vi "RFH-View-simple_common_selector.vi"() -> ()   [LabVIEW 2020, in "RFH-Reflection_File_Handler.lvlib"]
uses:
  RFH-Reflection_File_Handler.lvlib
panel:
  out "Reflection Imag 2":T1(graph)
  in  "stop":bool
  out "Numeric":i32
  out "Reflection Imag":T1(graph)
  in  "Folder Path":path=path "C:/projects/Universitet/Master/data/Real Test - First libreVNA test with calibration file/Converted Data"
  out "Reflection Real":T1(graph)
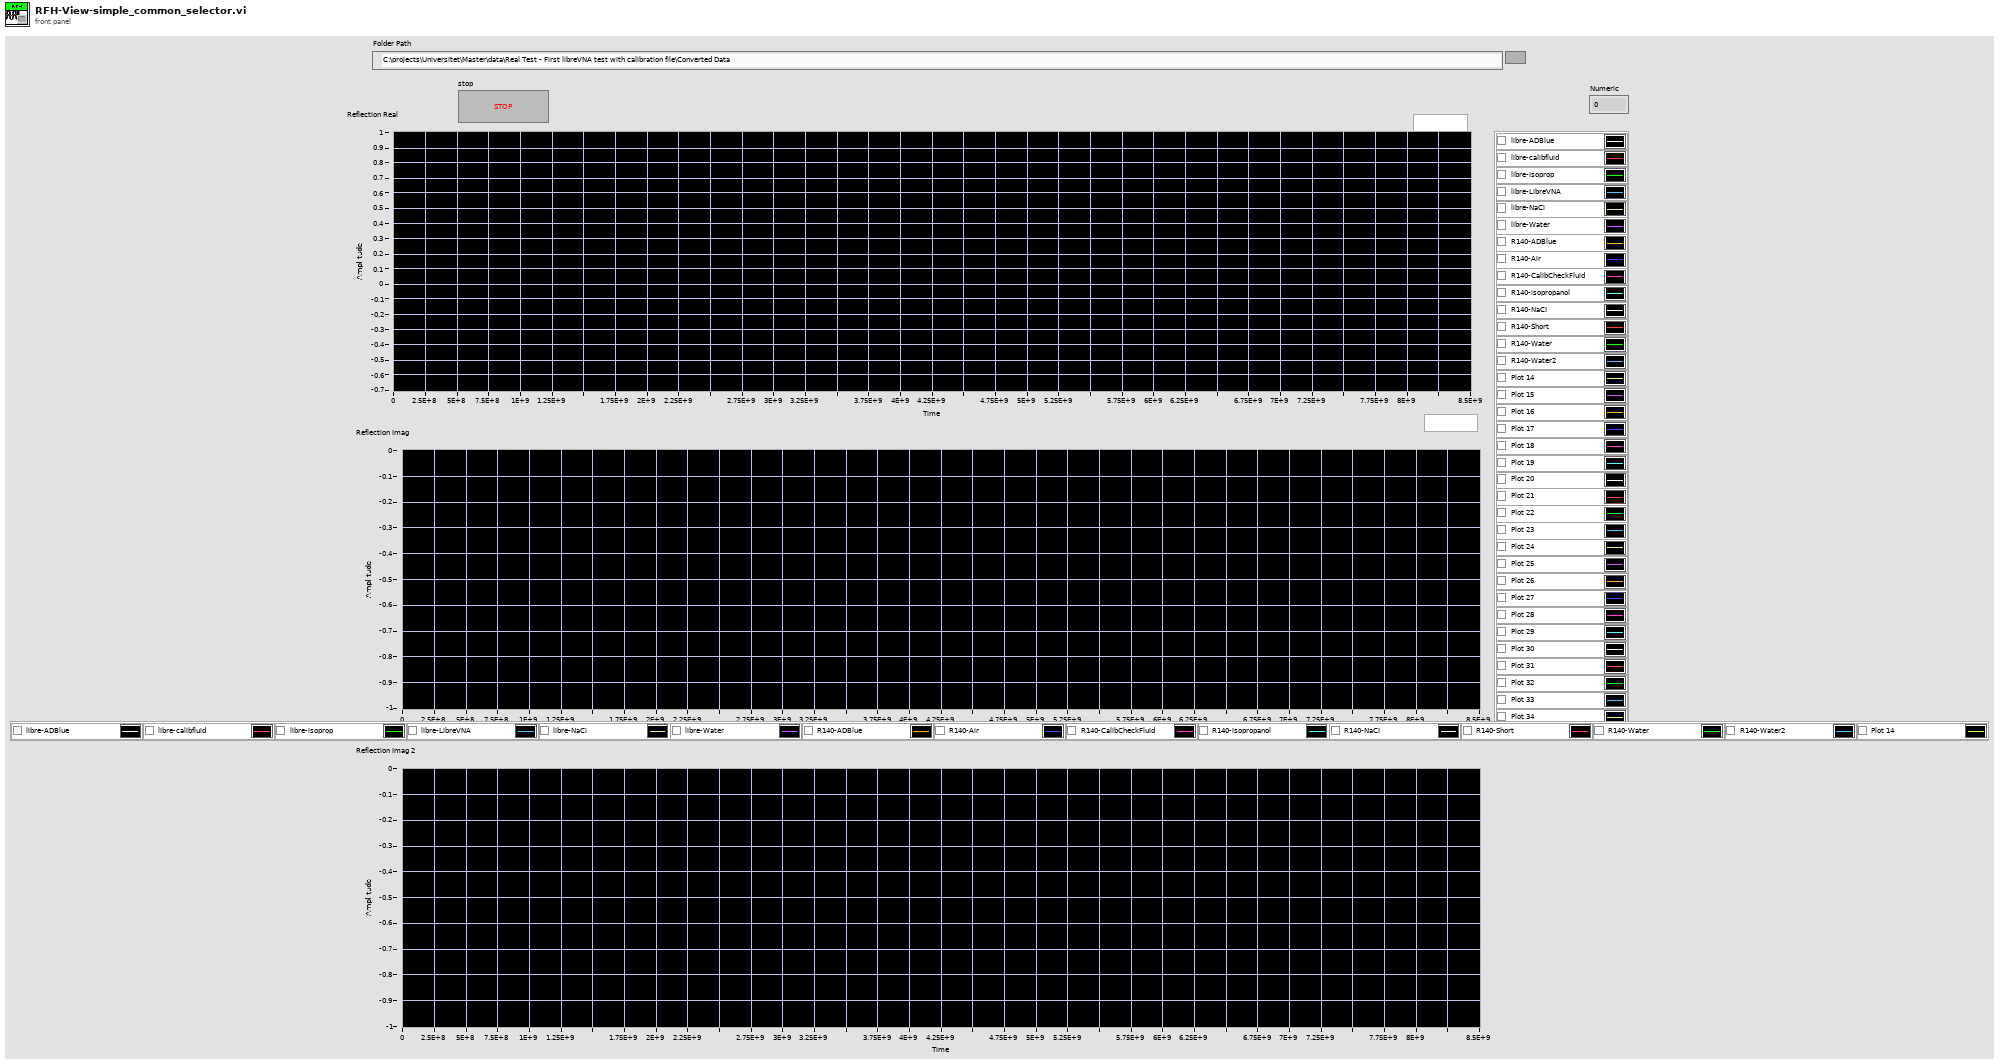
[diagram p1: front panel]
types:
  T1 = cluster{"Frequency":dbl[], "Reflection'":dbl[]}[]
  T2 = typedef "RFH-Reflection_File_Handler.lvlib/RFH-common_data_format.ctl" = cluster{"Frequency":dbl[], "Reflection'":dbl[], "Reflection''":dbl[], "Permativity'":dbl[], "Permativity''":dbl[]}
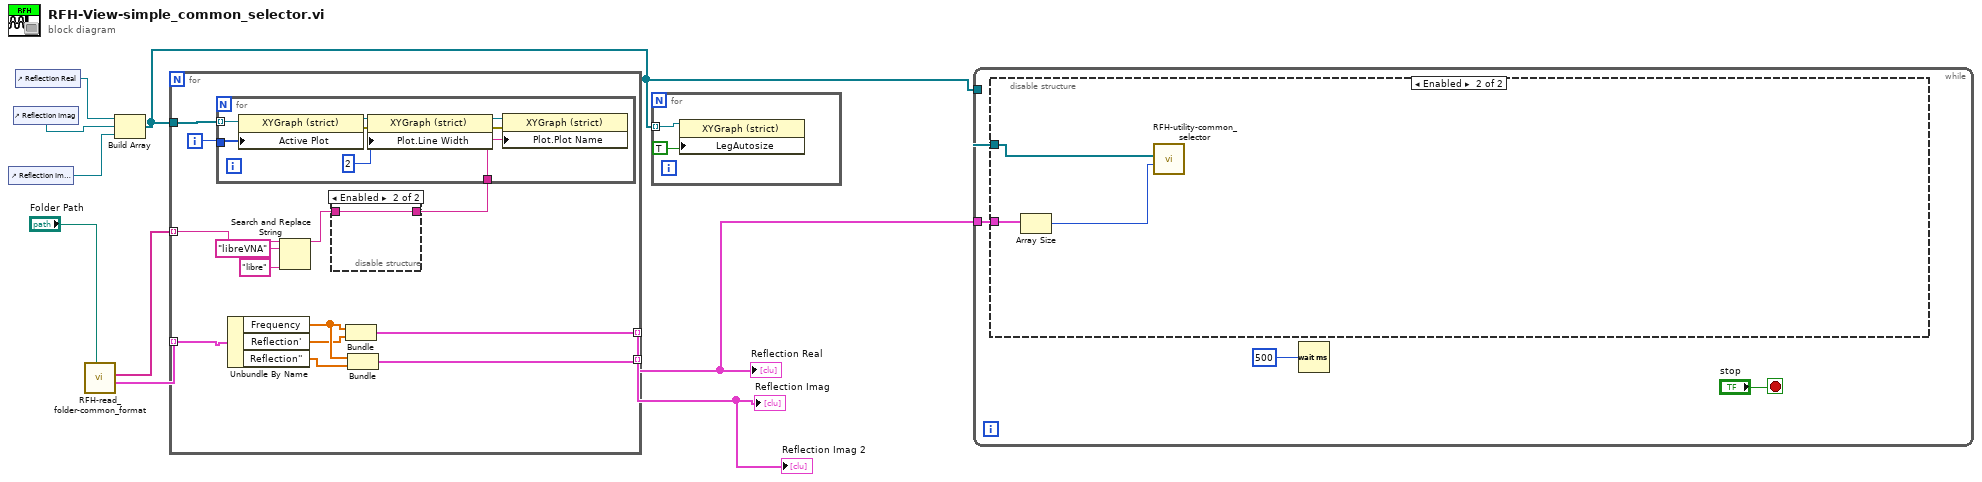
[diagram p0: block diagram]
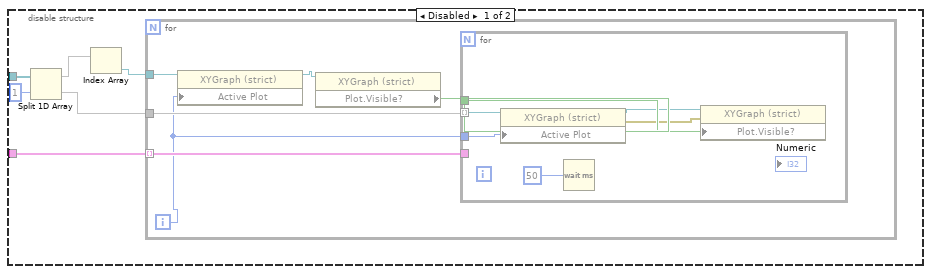
[diagram p2: hidden frame]
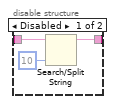
[diagram p3: hidden frame]
diagram:
  n1 = control-ref of="Reflection Imag 2"() -> (w4:refnum<vi>)
  n2 = control-ref of="Reflection Imag"() -> (w2:refnum<vi>)
  n3 = control-ref of="Reflection Real"() -> (w3:refnum<vi>)
  n4 = call "RFH-read_folder-common_format.vi"("Folder Path"="Folder Path") -> ("Data"=w9:T2[], "Names"=w7:string[])  [unwired: 8 in, 1 out]
  n5 = Build Array(w3, w2, w4) -> (w6:refnum<vi>[])
  n6 = for {
    tunnel: w9 -> [w22] mode=indexing
    tunnel: [w18] -> w1 mode=indexing
    tunnel: [w17] -> w5 mode=indexing
    tunnel: w7 -> [w14] mode=indexing
    tunnel: w6 -> [w10]
    i -> [w16]
    n7 = Unbundle By Name(w22) -> ("Frequency"=w21:dbl[], "Reflection'"=w20:dbl[], "Reflection''"=w19:dbl[])
    n8 = Search and Replace String(input string=w14, search string="libreVNA", replace string="libre" ("replace string (\"\")")) -> (result string=w11:string)  [unwired: 5 in, 3 out]
    n9 = disable-structure shown="Enabled" {
      disable-tunnel: [w24 w26] -> w15
      disable-tunnel: w11 -> [w23 w26]
      frame Disabled {
        n10 = Search/Split String(string=w23, offset (0)=10) -> (substring before match=w24:string)  [unwired: 1 in, 2 out]
      }
      frame Enabled {
      }
    }
    n11 = for {
      tunnel: w16 -> [w33]
      tunnel: w15 -> [w30]
      tunnel: w10 -> [w29] mode=indexing
      n12 = property on="Property Node" class="XYGraph (strict)"(reference=w29, "Active Plot"=w33) -> (reference out=w28:refnum<vi>, error out=w34:errorcluster)  [unwired: 1 in]
      n13 = property on="Property Node" class="XYGraph (strict)"(reference=w28, error in=w34, "Plot.Line Width"=u8 2) -> (reference out=w27:refnum<vi>, error out=w32:errorcluster)
      n14 = property on="Property Node" class="XYGraph (strict)"(reference=w27, error in=w32, "Plot.Plot Name"=w30) -> ()  [unwired: 2 out]
    }
    n15 = Bundle("Frequency"=w21, "Reflection'"=w20) -> (w18:cluster{"Frequency":dbl[], "Reflection'":dbl[]})  [unwired: 1 in]
    n16 = Bundle("Frequency"=w21, "Reflection''"=w19) -> (w17:cluster{"Frequency":dbl[], "Reflection''":dbl[]})  [unwired: 1 in]
  }
  "Reflection Real" <- w1
  "Reflection Imag" <- w5
  "Reflection Imag 2" <- w5
  n17 = for {
    tunnel: w6 -> [w35] mode=indexing
    n18 = property on="Property Node" class="XYGraph (strict)"(reference=w35, "LegAutosize"=TRUE ("Legend:Autosize")) -> ()  [unwired: 1 in, 2 out]
  }
  n19 = while {
    tunnel: w6 -> [w40]
    tunnel: w1 -> [w38]
    stop <- "stop" stop-if-true
    n20 = disable-structure shown="Enabled" {
      disable-tunnel: w40 -> [w46 w61]
      disable-tunnel: w38 -> [w42 w60]
      frame Disabled {
        n21 = Split 1D Array(array=w46, index=1) -> (first subarray=w44:refnum<vi>[], second subarray=w43:refnum<vi>[])
        n22 = Index Array(array=w44) -> (element=w41:refnum<vi>)  [unwired: 1 in]
        n23 = for {
          tunnel: w43 -> [w52]
          tunnel: w42 -> [w50] mode=indexing
          tunnel: w41 -> [w49]
          i -> [w47]
          n24 = property on="Property Node" class="XYGraph (strict)"(reference=w49, "Active Plot"=w47) -> (reference out=w48:refnum<vi>)  [unwired: 1 in, 1 out]
          n25 = property on="Property Node" class="XYGraph (strict)"(reference=w48) -> ("Plot.Visible?"=w51:bool)  [unwired: 1 in, 2 out]
          n26 = for {
            tunnel: w51 -> [w58]
            tunnel: w52 -> [w57] mode=indexing
            tunnel: w50 -> [_]
            tunnel: w47 -> [w53]
            n27 = property on="Property Node" class="XYGraph (strict)"(reference=w57, "Active Plot"=w53) -> (reference out=w56:refnum<vi>, error out=w55:errorcluster)  [unwired: 1 in]
            n28 = Wait (ms)(milliseconds to wait=u32 50) -> ()  [unwired: 1 out]
            n29 = property on="Property Node" class="XYGraph (strict)"(reference=w56, error in=w55, "Plot.Visible?"=w58) -> ()  [unwired: 2 out]
          }
        }
      }
      frame Enabled {
        n30 = Array Size(array=w60) -> (size(s)=w59:i32)
        n31 = call "RFH-utility-common_selector.vi"("size(s)"=w59, "XY graph refs"=w61) -> ()  [unwired: 10 in]
      }
    }
    n32 = Wait (ms)(milliseconds to wait=u32 500) -> ()  [unwired: 1 out]
  }
